vi "Complete.vi"   [LabVIEW 2015]
uses:
  class/Car.lvclass
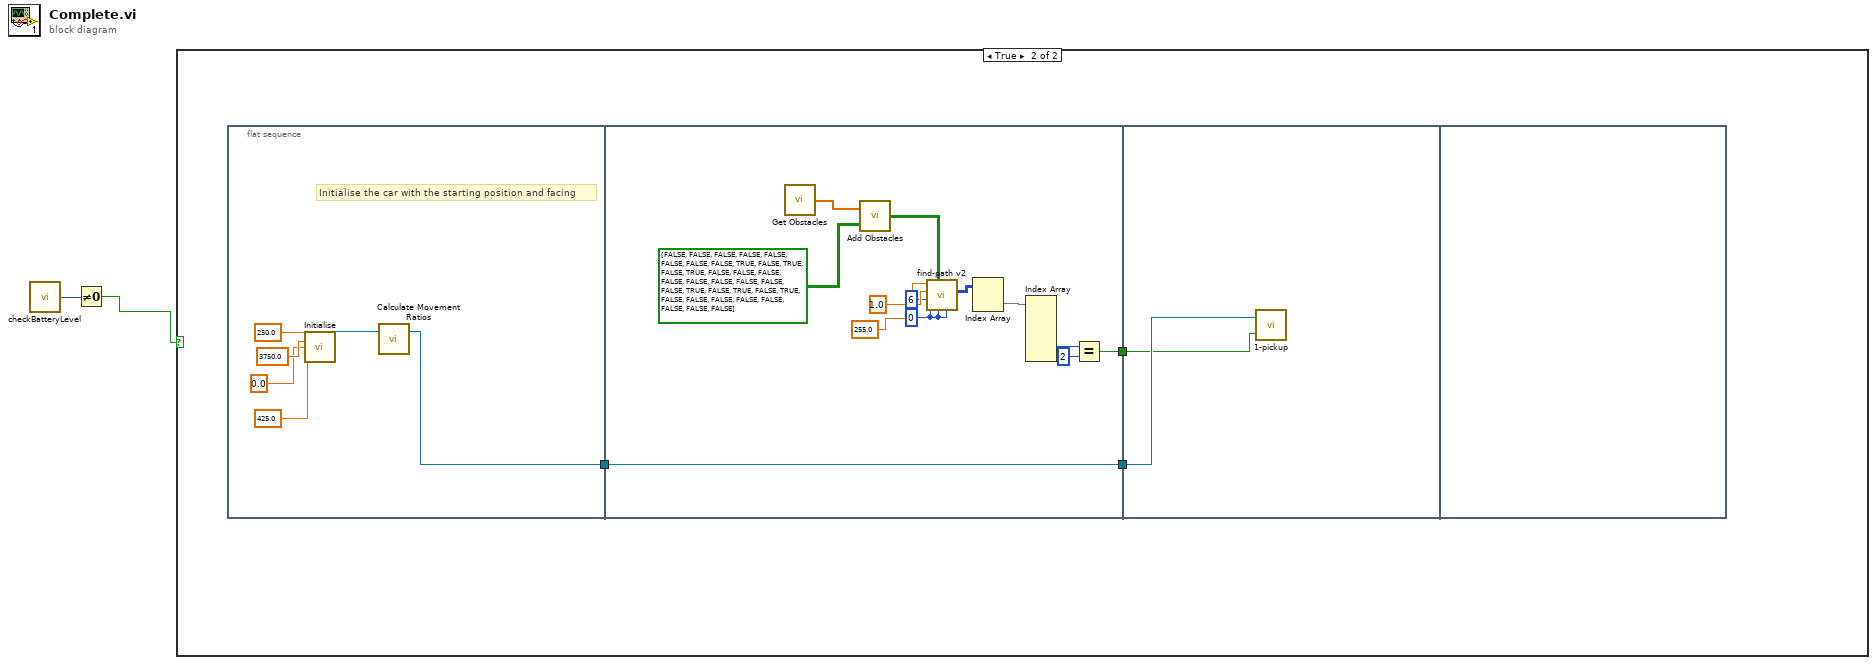
[diagram p0: block diagram]
diagram:
  n1 = call "checkBatteryLevel.vi"() -> ("Battery State"=w2:i32)
  n2 = Not Equal To 0?(x=w2) -> (x != 0?=w1:bool)
  n3 = case shown="True" w1 {
    frame False {
    }
    frame True {
      n4 = flat-sequence {
        tunnel: [w6] -> w5
        tunnel: w5 -> [w13]
        tunnel: [w13] -> w4
        tunnel: [w12] -> w3
        tunnel: w4 -> [w26]
        tunnel: w3 -> [w25]
        frame #0 {
          # "Initialise the car with the starting position and facing"
          n5 = call "Initialise.vi"("X"=250.0, "Y"=3750.0, "Facing"=0.0, "Size"=425.0) -> ("Car.lvclass"=w7:refnum<class "Car.lvclass">)  [unwired: 10 in, 1 out]
          n6 = call "Calculate Movement Ratios.vi"("Car.lvclass"=w7) -> ("Car.lvclass 2"=w6:refnum<class "Car.lvclass">)  [unwired: 1 in, 1 out]
        }
        frame #1 {
          w18 = i16 0 ("Destination Y")
          n7 = call "Get Obstacles.vi"() -> ("Obstacles"=w23:dbl[])
          n8 = call "Add Obstacles.vi"("Map"=bool[][] [[FALSE, FALSE, FALSE, FALSE, FALSE, FALSE, FALSE], [FALSE, TRUE, FALSE, TRUE, FALSE, TRUE, FALSE], [FALSE, FALSE, FALSE, FALSE, FALSE, FALSE, FALSE], [FALSE, TRUE, FALSE, TRUE, FALSE, TRUE, FALSE], [FALSE, FALSE, FALSE, FALSE, FALSE, FALSE, FALSE]], "Obstacles"=w23) -> ("Map With Obstacles"=w22:bool[][])
          n9 = call "find-path v2.vi"("Start Y"=w18, "Start X"=w18, "Obstacles"=w22, "Destination Y"=w18, "Destination X"=i16 6, "Empty Value"=1.0, "Wall Value"=255.0 ("Wall value")) -> ("Instructions"=w17:i32[][])  [unwired: 3 in, 1 out]
          n10 = Index Array(array=w17) -> (element=w16:i32[])  [unwired: 2 in]
          n11 = Index Array(array=w16) -> (element #5=w15:i32)  [unwired: 6 in, 5 out]
          n12 = Equal?(x=w15, y=2) -> (x = y?=w12:bool)
        }
        frame #2 {
          n13 = call "1-pickup.vi"("U-Turn?"=w25, "Car.lvclass"=w26) -> ()  [unwired: 1 in]
        }
        frame #3 {
        }
      }
    }
  }
